vi "Air MFR sw 1.vi"(10 "C_air":dbl, 11 "Flow rate":dbl) -> (3 "Air MFR":dbl)   [LabVIEW 2014]
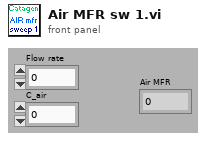
[diagram p1: front panel]
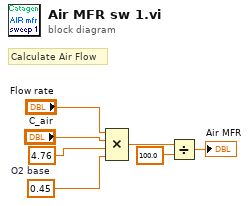
[diagram p0: block diagram]
diagram:
  w1 = 0.45  # O2 base
  # "Calculate Air Flow"
  n1 = Compound Arithmetic op=MULTIPLY("Flow rate", "C_air", 4.76, w1) -> (w5:dbl)
  n2 = Divide(x=w5, y=100.0) -> (x/y=→"Air MFR":dbl)
